vi "Copie de Init_graphe.vi"() -> ()   [LabVIEW 2013]
uses:
  <vilib>/Utility/miscctls.llb/LVRowAndColumnTypeDef.ctl
  <vilib>/Utility/file.llb/Read From Spreadsheet File (string).vi
panel:
  in  "Horodatage":timestamp
  in  "Bouton Aide":bool
  in  "Quit":bool
  out "horodatage_ok":timestamp
  in  "Fichier données":path
  out "Colonne données brutes":string="0"
  out "Ligne données brutes":string="0"
  out "Noms variables":string[](array[string])
  out "Séparateur fichier brute":string
  in  "Valider":bool
  in  "Nouveau format date":bool
  in  "Format d'horodatage":string(combo)="\"%Y-%m-%d %H:%M:%S\""
  in  "Convertir Horodatage":bool
  out "Nb lignes":i32
  in  "Séparateur":u16(ring)=1 items=["", ",", ";", ".", "Tab", "Espace", ":"]
  out "Horodatage_1":timestamp[](array[timestamp]) format="%<%X\n%x>T"
  out "Table":string[][](table)
  out "Donnees":dbl[][](array[numeric])
  in  "Bouton vide 2":bool
  # "Facultatif : \nSélectionner la dernière cellule des noms de variables  en appuyant sur la touche CTRL"
  # "Sélectionner la 1ère cellule\ndes noms de variables"
  # "Sélectionner la 1ère cellule\nd'horodatage"
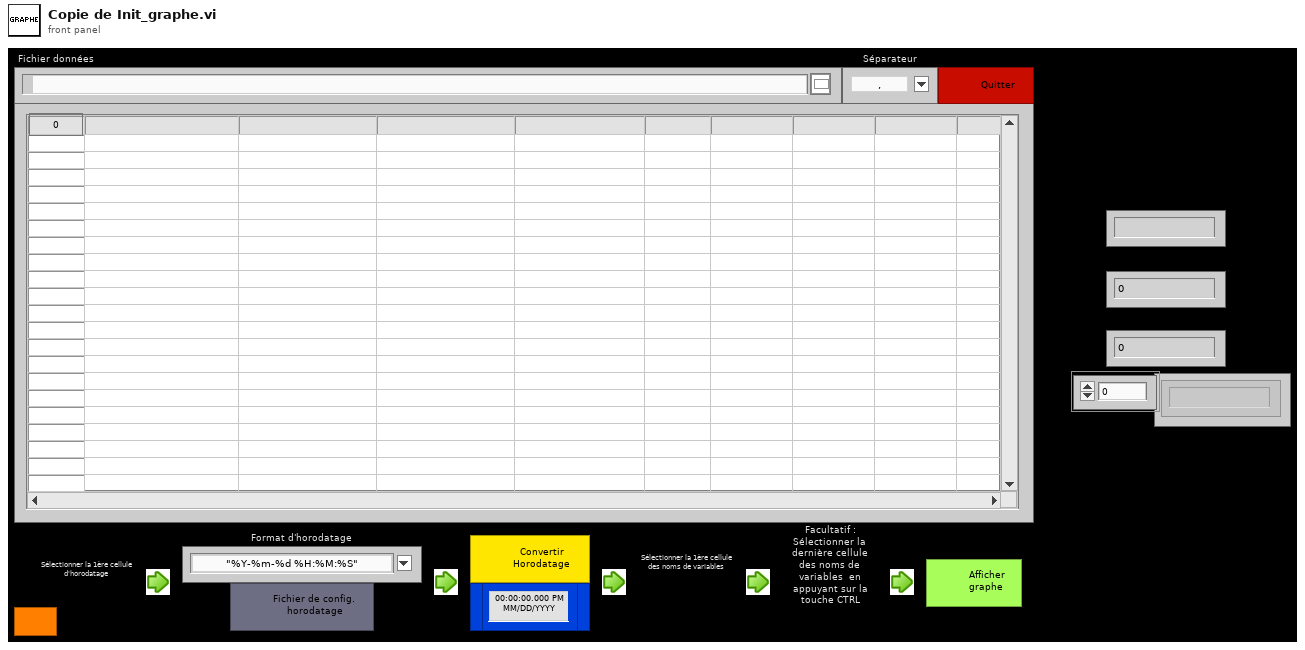
[diagram p1: front panel]
types:
  T1 = typedef "LVRowAndColumnTypeDef.ctl" = cluster{"Row":i32, "Column":i32}
  T2 = typedef "excel Object Reference.ctl" = refnum<k1>
  T3 = enum16{"Left Button", "Center Button", "Right Button", "Window Close"}
  T4 = cluster{"Shift":bool, "Ctrl":bool, "Alt":bool, "Cmd":bool, "Opt":bool}
  T5 = cluster{"Horodatage":timestamp[], "Donnees":dbl[]}[]
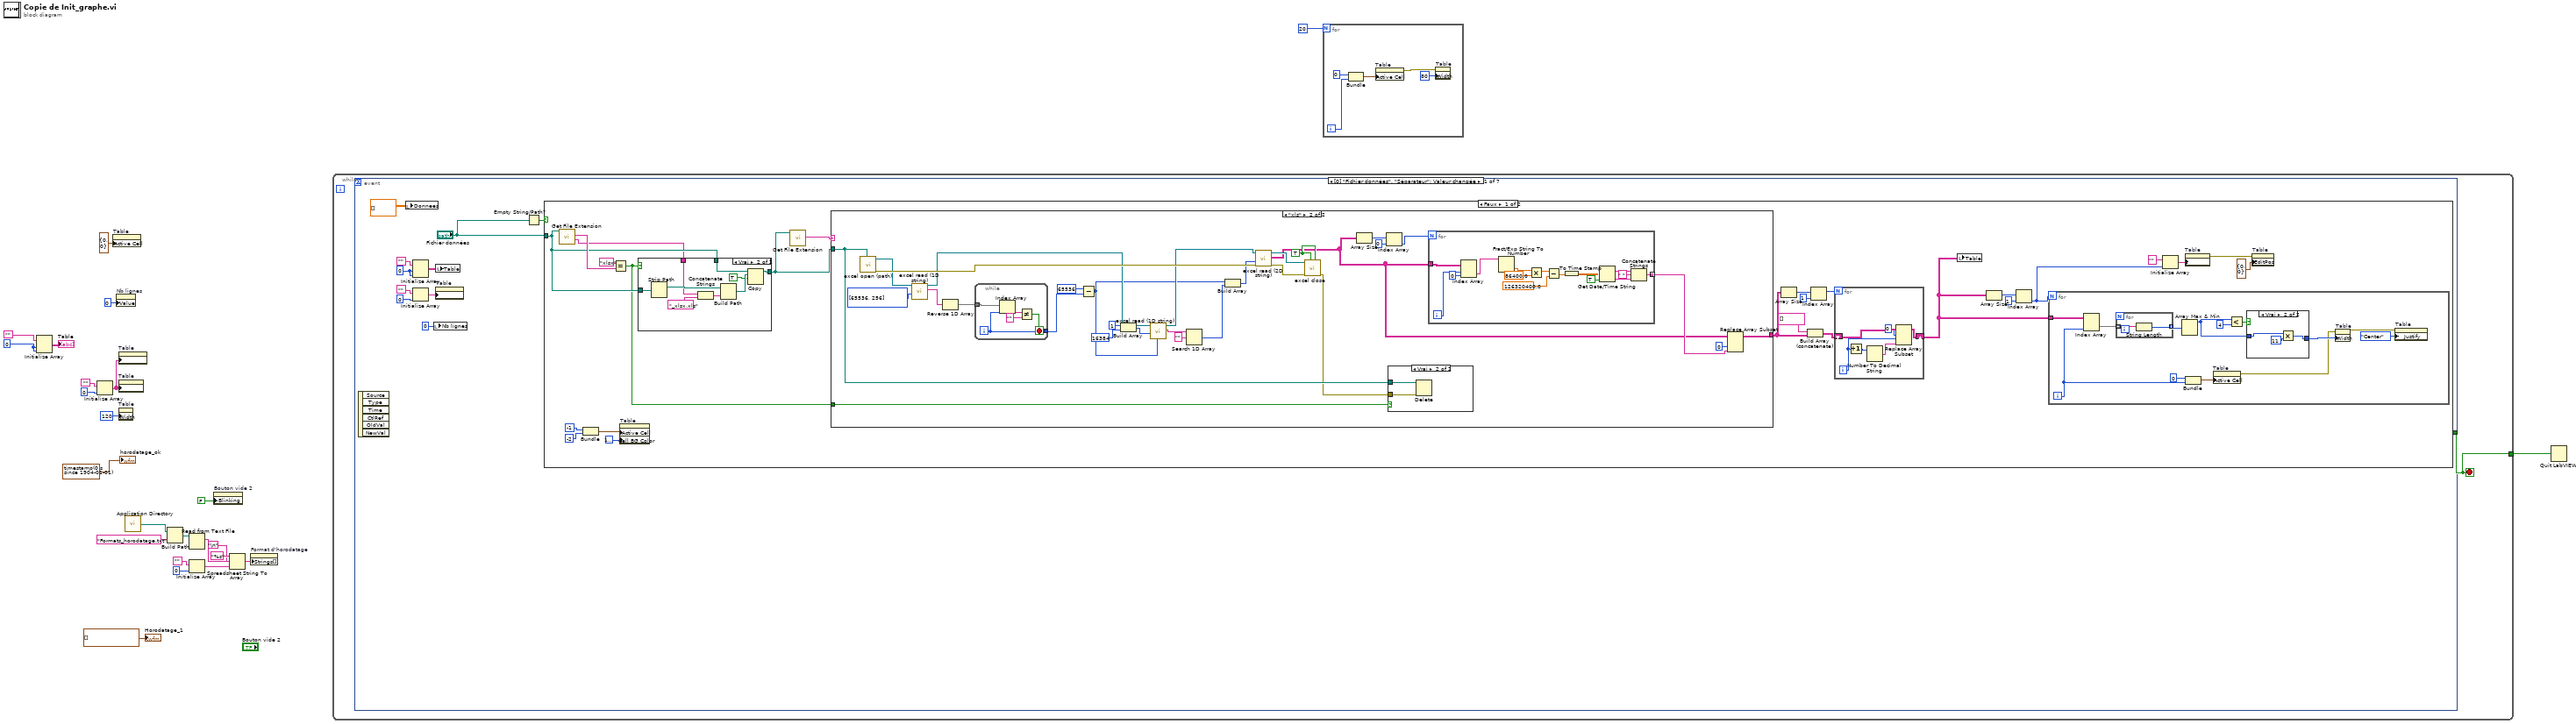
[diagram p0: block diagram]
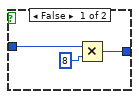
[diagram p3: hidden frame]
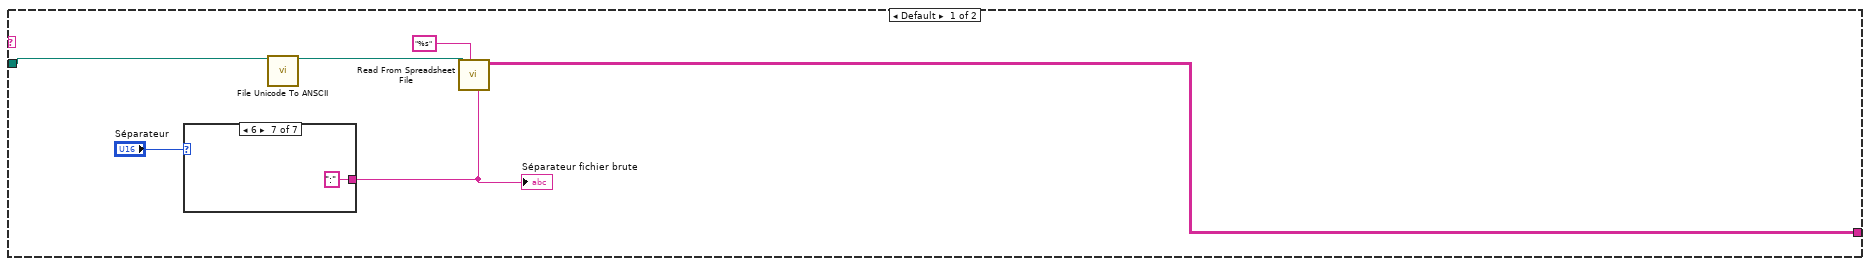
[diagram p4: hidden frame]
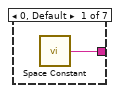
[diagram p5: hidden frame]
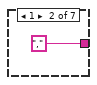
[diagram p6: hidden frame]
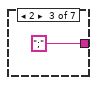
[diagram p7: hidden frame]
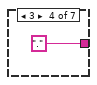
[diagram p8: hidden frame]
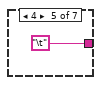
[diagram p9: hidden frame]
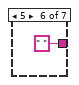
[diagram p10: hidden frame]
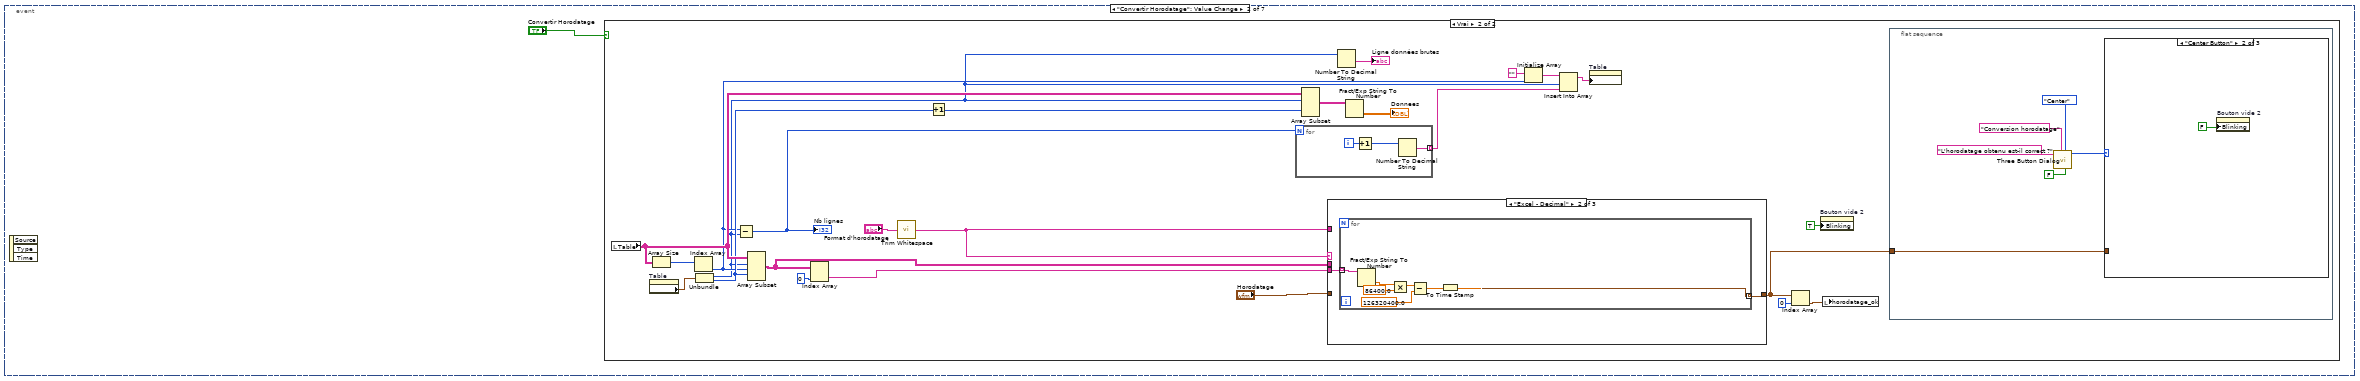
[diagram p13: hidden frame]
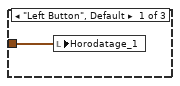
[diagram p15: hidden frame]
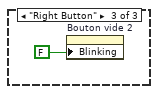
[diagram p16: hidden frame]
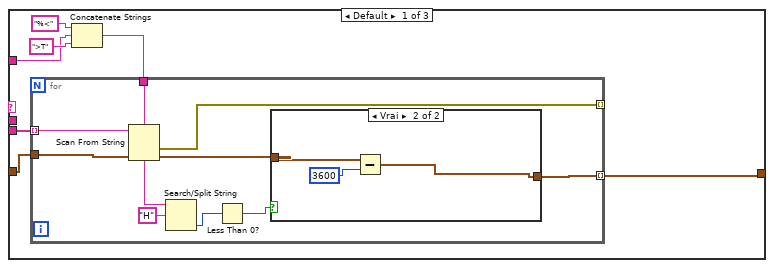
[diagram p17: hidden frame]
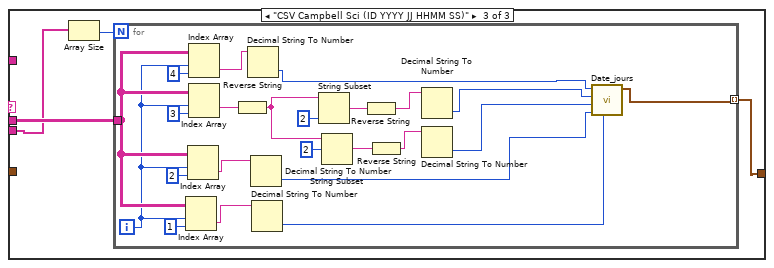
[diagram p19: hidden frame]
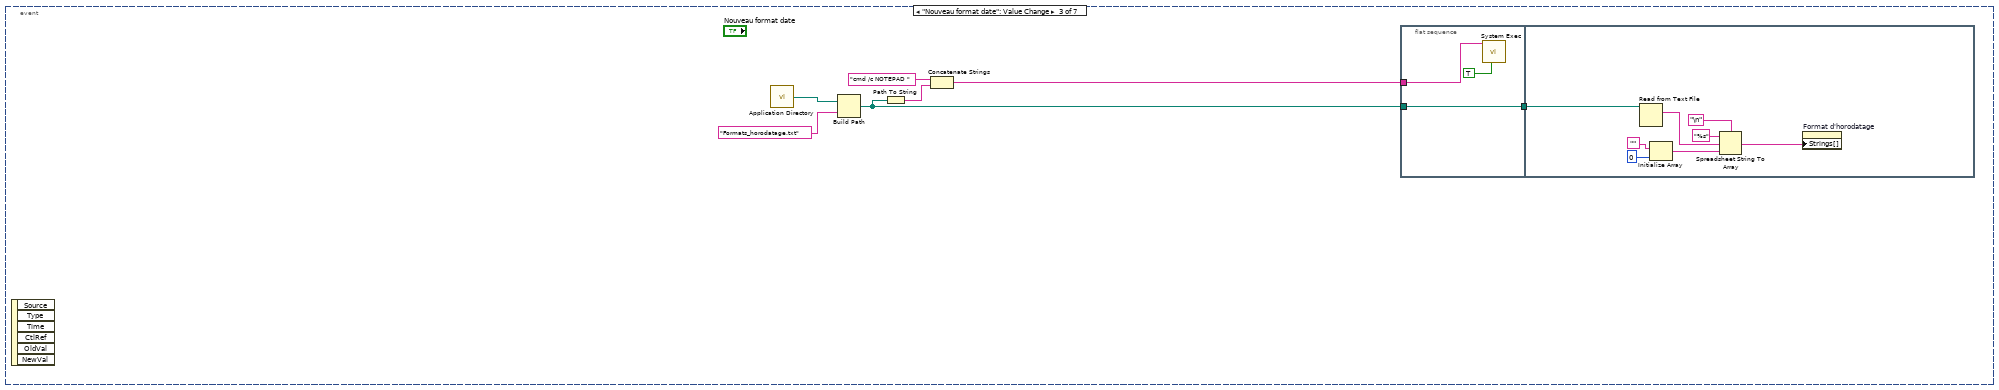
[diagram p20: hidden frame]
diagram:
  w6 = 0 ("taille de la dimension")
  n1 = Initialize Array("", w6, w6) -> (→"Table":string[][])
  n2 = Initialize Array("", 0 ("taille de la dimension")) -> (w13:string[])
  n3 = property on="Table" class="Tbl (strict)"("Active Cell"=T1 {"Row"=0, "Column"=0} ("Cellule active:Cellule active")) -> ()  [unwired: 2 in, 2 out]
  n4 = property on="Nb lignes" class="NumNb (strict)"("Value"=0 ("Nb lignes")) -> ()  [unwired: 2 in, 2 out]
  n5 = property on="Table" class="Tbl (strict)"("Row Headers[]"=w13) -> ()  [unwired: 2 in, 2 out]
  n6 = property on="Table" class="Tbl (strict)"("Column Headers[]"=w13) -> ()  [unwired: 2 in, 2 out]
  n7 = property on="Table" class="Tbl (strict)"("Width"=u32 120 ("Cellule active:Taille de la cellule:Largeur")) -> ()  [unwired: 2 in, 2 out]
  n8 = call <vilib>:"Application Directory.vi"() -> ("Application Directory"=w9:path)
  n9 = Build Path(base path=w9, name or relative path="Formats_horodatage.txt" ("nom ou chemin relatif")) -> (appended path=w17:path)
  n10 = Read from Text File(file (use dialog)=w17) -> (text=w22:string)  [unwired: 3 in, 3 out]
  n11 = Initialize Array("", 0 ("taille de la dimension")) -> (w18:string[])
  n12 = property on="Bouton vide 2" class="Bool"("Blinking"=FALSE ("Clignotant")) -> ()  [unwired: 2 in, 2 out]
  n13 = Spreadsheet String To Array(delimiter (Tab)="\n", format string="%s" ("chaîne de format"), spreadsheet string=w22, array type (2D Dbl)=w18) -> (array=w14:string[])
  n14 = property on="Format d'horodatage" class="ChneDér"("Strings[]"=w14) -> ()  [unwired: 2 in, 2 out]
  n15 = while {
    tunnel: [w25] -> w3
    stop <- w25 stop-if-true
    n16 = event shown="[0] \"Fichier données\", \"Séparateur\": Valeur changée" {
      selector: _ -> [_ _ _ _ _ _ _]
      dyn-events: _ -> [_ _ _ _ _ _ _]
      timeout: _ -> [_ _ _ _ _ _ _]
      tunnel: [_ _ _ _ _ w377 _] -> w25
      event "Fichier données", "Séparateur": Value Change {
        w35 = 0 ("taille de la dimension")
        n17 = event-data() -> ()  [unwired: 1 in, 6 out]
        n18 = local write "Donnees"(dbl[][] [] ("Donnees")) -> ()
        n19 = Initialize Array("", w35, w35) -> (w33:string[][])
        n20 = Initialize Array("", 0 ("taille de la dimension")) -> (w30:string[])
        n21 = local write "Nb lignes"(0 ("Nb lignes")) -> ()
        n22 = local write "Table"(w33) -> ()
        n23 = property on="Table" class="Tbl (strict)"("Row Headers[]"=w30) -> ()  [unwired: 2 in, 2 out]
        n24 = Empty String/Path?(string/path="Fichier données") -> (empty?=w27:bool)
        n25 = case shown="Faux" w27 {
          tunnel: "Fichier données" -> [w40 _]
          frame False {
            n26 = call <vilib>:"Get File Extension.vi"("file"=w40) -> ("filename without extension"=w39:string, "lowercase file extension"=w42:string)  [unwired: 7 in, 2 out]
            n27 = Bundle(-1, -2) -> (w53:cluster{i32, i32})  [unwired: 1 in]
            n28 = Equal?(x="xlsx", y=w42) -> (x = y?=w36:bool)
            n29 = property on="Table" class="Tbl (strict)"("Active Cell"=w53, "Cell BG Color"=u32 16777225) -> ()  [unwired: 2 in, 2 out]
            n30 = case shown="Vrai" w36 {
              tunnel: w40 -> [w61 w70]
              tunnel: [w61 w69] -> w38
              tunnel: w40 -> [_ w67]
              tunnel: w39 -> [_ w64]
              frame False {
              }
              frame True {
                n31 = Strip Path(path=w67) -> (stripped path=w68:path)  [unwired: 1 out]
                n32 = Concatenate Strings(w64, "_xlsx.xls" ("chaîne")) -> (w65:string)
                n33 = Build Path(base path=w68, name or relative path=w65) -> (appended path=w66:path)
                n34 = Copy(9:TRUE ("écraser (F)"), 10:w66, 11:w70) -> (3:w69:path)  [unwired: 2 in, 2 out]
              }
            }
            n35 = call <vilib>:"Get File Extension.vi"("file"=w38) -> ("lowercase file extension"=w37:string)  [unwired: 7 in, 3 out]
            n36 = case shown="\"xls\"" w37 {
              tunnel: w38 -> [w99 w113]
              tunnel: [w101 w114] -> w46
              tunnel: w36 -> [_ w111]
              frame Default {
                n37 = case shown="6" "Séparateur" {
                  tunnel: [w104 "," ";" "." "\t" " " ("String") ":" ("String")] -> w100
                  frame 0, Default {
                    n38 = call <vilib>:"Space Constant.vi"() -> ("String"=w104:string)
                  }
                  frame 1 {
                  }
                  frame 2 {
                  }
                  frame 3 {
                  }
                  frame 4 {
                  }
                  frame 5 {
                  }
                  frame 6 {
                  }
                }
                "Séparateur fichier brute" <- w100
                n39 = call "File Unicode To ANSCII.vi"("file in"=w99) -> ("file out"=w98:path)  [unwired: 18 in]
                n40 = call-poly <vilib>:"Read From Spreadsheet File.vi"("delimiter (\\t)"=w100, "format (%s)"="%s", "file path (dialog if empty)"=w98) -> ("all rows"=w101:string[][])  [unwired: 4 in, 4 out]
              }
              frame "xls" {
                w137 = TRUE ("Override closing behavior")
                n41 = call <userlib>:"excel open (path).vi"("workbook path"=w113) -> ("error out"=w138:errorcluster, "reference"=w136:T2)  [unwired: 9 in]
                n42 = call <userlib>:"excel read (1D string).vi"("array size\n  - #rows\n  - #columns"=i32[] [65536, 256] ("array size\n  - #rows\n  - #columns"), "reference"=w136) -> ("1D String Array"=w134:string[], "duplicate reference"=w127:T2)  [unwired: 7 in, 1 out]
                n43 = Reverse 1D Array(array=w134) -> (reversed array=w132:string[])
                n44 = while {
                  tunnel: w132 -> [w162]
                  tunnel: [w158] -> w131
                  i -> [w158]
                  stop <- w159 stop-if-true
                  n45 = Index Array(array=w162, index=w158) -> (element=w161:string)
                  n46 = Not Equal?(x=w161, y="") -> (x != y?=w159:bool)
                }
                n47 = Subtract(x=65536, y=w131) -> (x-y=w124:i32)
                n48 = Build Array(1 ("élément"), 16384 ("élément")) -> (w128:i32[])
                n49 = call <userlib>:"excel read (1D string).vi"("Row"=w124, "array size\n  - #rows\n  - #columns"=w128, "reference"=w127) -> ("1D String Array"=w123:string[], "duplicate reference"=w126:T2)  [unwired: 6 in, 1 out]
                n50 = Search 1D Array(1D array=w123, element="" ("élément")) -> (index of element=w121:i32)  [unwired: 1 in]
                n51 = Build Array(w124, w121) -> (w133:i32[])
                n52 = call <userlib>:"excel read (2D string).vi"("error in (no error)"=w138, "array size\n  - #rows\n  - #columns"=w133, "reference"=w126) -> ("error out"=w139:errorcluster, "2D String Array"=w115:string[][], "duplicate reference"=w140:T2)  [unwired: 6 in]
                n53 = call <userlib>:"excel close.vi"("Close"=w137, "Override closing behavior"=w137, "error in (no error)"=w139, "reference"=w140) -> ("error out"=w112:errorcluster)  [unwired: 7 in]
                n54 = Array Size(array=w115) -> (size(s)=w117:i32[])
                n55 = Index Array(array=w117, index=0 ("indice")) -> (element=w118:i32)
                n56 = case shown="Vrai" w111 {
                  tunnel: w113 -> [_ w142]
                  tunnel: w112 -> [_ w141]
                  frame False {
                  }
                  frame True {
                    n57 = Delete(path (use dialog)=w142, error in=w141) -> ()  [unwired: 3 in, 3 out]
                  }
                }
                n58 = for {
                  N: w118 -> [_]
                  tunnel: w115 -> [w157]
                  tunnel: [w143] -> w120 mode=indexing
                  i -> [w156]
                  n59 = Index Array(array=w157, index (row)=w156, index (col)=0 ("indice désactivé (col)")) -> (element=w144:string)
                  n60 = Fract/Exp String To Number(string=w144) -> (number=w154:dbl)  [unwired: 3 in, 1 out]
                  n61 = Multiply(x=w154, y=86400.0) -> (x*y=w152:dbl)
                  n62 = Subtract(x=w152, y=126320400.0) -> (x-y=w150:dbl)
                  n63 = To Time Stamp(1:w150) -> (0:w149:timestamp)
                  n64 = Get Date/Time String(seconds (now)=w149, want seconds? (F)=TRUE ("secondes ? (F)")) -> (date string=w147:string, time string=w145:string)  [unwired: 1 in]
                  n65 = Concatenate Strings(w147, " " ("chaîne"), w145) -> (w143:string)
                }
                n66 = Replace Array Subset(array=w115, new element=w120, index (col)=0 ("indice désactivé (col)")) -> (w114:string[][])  [unwired: 1 in]
              }
            }
            n67 = Array Size(array=w46) -> (size(s)=w48:i32[])
            n68 = Build Array (concatenate)(string[] [] ("élément"), w46) -> (w44:string[][])
            n69 = Index Array(array=w48, index=1 ("indice")) -> (element=w47:i32)
            n70 = for {
              N: w47 -> [_]
              shift-right: [w76] -> w50
              shift-left: w44 -> [w75]
              i -> [w72]
              n71 = Increment(x=w72) -> (x+1=w74:i32)
              n72 = Number To Decimal String(number=w74) -> (decimal integer string=w71:string)  [unwired: 1 in]
              n73 = Replace Array Subset(array=w75, new element=w71, index (row)=0 ("indice désactivé (ligne)"), index (col)=w72) -> (w76:string[][])
            }
            n74 = local write "Table"(w50) -> ()
            n75 = Array Size(array=w50) -> (size(s)=w56:i32[])
            n76 = Index Array(array=w56, index=1 ("indice")) -> (element=w43:i32)
            n77 = for {
              N: w43 -> [_]
              tunnel: w50 -> [w89]
              i -> [w83]
              n78 = Index Array(array=w89, index (col)=w83) -> (element=w87:string[])  [unwired: 1 in]
              n79 = for {
                tunnel: w87 -> [w97] mode=indexing
                tunnel: [w96] -> w86 mode=indexing
                n80 = String Length(string=w97) -> (length=w96:i32)
              }
              n81 = Array Max & Min(array=w86) -> (max value=w78:i32)  [unwired: 3 out]
              n82 = Bundle(0, w83) -> (w85:cluster{i32, i32})  [unwired: 1 in]
              n83 = property on="Table" class="Tbl (strict)"("Active Cell"=w85) -> (error out=w84:errorcluster)  [unwired: 2 in, 1 out]
              n84 = Less?(x=w78, y=4) -> (x < y?=w79:bool)
              n85 = case shown="Vrai" w79 {
                tunnel: [w92 w93] -> w88
                tunnel: w78 -> [w90 w94]
                frame False {
                  n86 = Multiply(x=w90, y=8) -> (x*y=w92:i32)
                }
                frame True {
                  n87 = Multiply(x=w94, y=11) -> (x*y=w93:i32)
                }
              }
              n88 = property on="Table" class="Tbl (strict)"(error in=w84, "Width"=w88) -> (error out=w81:errorcluster)  [unwired: 1 in, 1 out]
              n89 = property on="Table" class="Tbl (strict)"(error in=w81, "Justify"=enum16{"Left", "Center", "Right"}."Center" ("Cellule active:Justification de la cellule")) -> ()  [unwired: 1 in, 2 out]
            }
            n90 = Initialize Array("", w43) -> (w59:string[])
            n91 = property on="Table" class="Tbl (strict)"("Column Headers[]"=w59) -> (error out=w57:errorcluster)  [unwired: 2 in, 1 out]
            n92 = property on="Table" class="Tbl (strict)"(error in=w57, "EditPos"=T1 {"Row"=0, "Column"=0} ("Cellule active:Cellule active")) -> ()  [unwired: 1 in, 2 out]
          }
          frame True {
          }
        }
      }
      event "Convertir Horodatage": Value Change {
        n93 = event-data() -> ()  [unwired: 1 in, 3 out]
        n94 = case shown="Vrai" "Convertir Horodatage" {
          frame False {
          }
          frame True {
            n95 = local read "Table"() -> (w183:string[][])
            n96 = property on="Table" class="Tbl (strict)"() -> ("Selection Start"=w186:T1)  [unwired: 2 in, 2 out]
            n97 = Array Size(array=w183) -> (size(s)=w184:i32[])
            n98 = Index Array(array=w184) -> (element=w178:i32)  [unwired: 1 in]
            n99 = Unbundle(w186) -> ("Row"=w174:i32, "Column"=w179:i32)
            n100 = Subtract(x=w178, y=w174) -> (x-y=w169:i32)
            "Nb lignes" <- w169
            n101 = Array Subset(array=w183, index (row)=w174, length (row)=w178, index (col)=w179) -> (w171:string[][])  [unwired: 1 in]
            n102 = Index Array(array=w171, index (col)=0 ("indice (ligne)")) -> (element=w176:string[])  [unwired: 1 in]
            n103 = call <vilib>:"Trim Whitespace.vi"("string"="Format d'horodatage") -> ("trimmed string"=w165:string)  [unwired: 1 in]
            n104 = Increment(x=w179) -> (x+1=w185:i32)
            n105 = for {
              N: w169 -> [_]
              tunnel: [w255] -> w180 mode=indexing
              i -> [w256]
              n106 = Increment(x=w256) -> (x+1=w254:i32)
              n107 = Number To Decimal String(number=w254) -> (decimal integer string=w255:string)  [unwired: 1 in]
            }
            n108 = Array Subset(array=w183, index (row)=w174, index (col)=w185) -> (w187:string[][])  [unwired: 2 in]
            n109 = case shown="\"Excel - Decimal\"" w165 {
              tunnel: "Horodatage" -> [w204 _ _]
              tunnel: w176 -> [w201 w219 w227]
              tunnel: [w200 w218 w229] -> w168
              tunnel: w165 -> [w198 _ _]
              tunnel: w171 -> [_ _ w230]
              frame Default {
                n110 = Concatenate Strings("%<", w198, ">T") -> (w199:string)
                n111 = for {
                  tunnel: [w208] -> w200 mode=indexing
                  tunnel: w204 -> [w213]
                  tunnel: w199 -> [w211]
                  tunnel: w201 -> [w212] mode=indexing
                  tunnel: [w205] -> _ mode=indexing
                  n112 = Scan From String(format string=w211, input string=w212, default 1=w213) -> (error out=w205:errorcluster, output 1=w209:timestamp)  [unwired: 2 in, 2 out]
                  n113 = Search/Split String(string=w211, search string/char (-)="H" ("chaîne/car. recherché (-)")) -> (offset of match=w207:i32)  [unwired: 1 in, 2 out]
                  n114 = Less Than 0?(x=w207) -> (x < 0?=w206:bool)
                  n115 = case shown="Vrai" w206 {
                    tunnel: w209 -> [w214 w217]
                    tunnel: [w214 w215] -> w208
                    frame False {
                    }
                    frame True {
                      n116 = Subtract(x=w217, y=3600) -> (x-y=w215:timestamp)
                    }
                  }
                }
              }
              frame "Excel - Decimal" {
                n117 = for {
                  tunnel: [w220] -> w218 mode=indexing
                  tunnel: w219 -> [w226] mode=indexing
                  n118 = Fract/Exp String To Number(string=w226) -> (number=w225:dbl)  [unwired: 3 in, 1 out]
                  n119 = Multiply(x=w225, y=86400.0) -> (x*y=w223:dbl)
                  n120 = Subtract(x=w223, y=126320400.0) -> (x-y=w221:dbl)
                  n121 = To Time Stamp(1:w221) -> (0:w220:timestamp)
                }
              }
              frame "CSV Campbell Sci (ID YYYY JJ HHMM SS)" {
                n122 = Array Size(array=w227) -> (size(s)=w228:i32)
                n123 = for {
                  N: w228 -> [_]
                  tunnel: w230 -> [w240]
                  tunnel: [w231] -> w229 mode=indexing
                  i -> [w239]
                  n124 = Index Array(array=w240, index (row)=w239, index (col)=1 ("indice désactivé (col)")) -> (element=w237:string)
                  n125 = Index Array(array=w240, index (row)=w239, index (col)=2 ("indice désactivé (col)")) -> (element=w238:string)
                  n126 = Index Array(array=w240, index (row)=w239, index (col)=4 ("indice désactivé (col)")) -> (element=w252:string)
                  n127 = Index Array(array=w240, index (row)=w239, index (col)=3 ("indice désactivé (col)")) -> (element=w250:string)
                  n128 = Reverse String(1:w250) -> (0:w246:string)
                  n129 = Decimal String To Number(string=w252) -> (number=w236:i32)  [unwired: 2 in, 1 out]
                  n130 = Decimal String To Number(string=w238) -> (number=w233:i32)  [unwired: 2 in, 1 out]
                  n131 = Decimal String To Number(string=w237) -> (number=w232:i32)  [unwired: 2 in, 1 out]
                  n132 = String Subset(string=w246, length (rest)=2 ("longueur (reste)")) -> (substring=w248:string)  [unwired: 1 in]
                  n133 = String Subset(string=w246, offset (0)=2) -> (substring=w244:string)  [unwired: 1 in]
                  n134 = Reverse String(1:w248) -> (0:w247:string)
                  n135 = Reverse String(1:w244) -> (0:w243:string)
                  n136 = Decimal String To Number(string=w247) -> (number=w235:i32)  [unwired: 2 in, 1 out]
                  n137 = Decimal String To Number(string=w243) -> (number=w234:i32)  [unwired: 2 in, 1 out]
                  n138 = call "Date_jours.vi"("year"=w232, "jours n"=w233, "hour"=w234, "minute"=w235, "second"=w236) -> ("horodatage"=w231:timestamp)  [unwired: 6 in]
                }
              }
            }
            n139 = Number To Decimal String(number=w174) -> (decimal integer string=→"Ligne données brutes":string)  [unwired: 1 in]
            n140 = Fract/Exp String To Number(string=w187) -> (number=→"Donnees":dbl[][])  [unwired: 3 in, 1 out]
            n141 = Initialize Array("", w178) -> (w181:string[])
            n142 = Insert Into Array(array=w181, index=w174, new element=w180) -> (w170:string[])
            n143 = property on="Table" class="Tbl (strict)"("Row Headers[]"=w170) -> ()  [unwired: 2 in, 2 out]
            n144 = Index Array(array=w168, index=0 ("indice")) -> (element=w167:timestamp)
            n145 = property on="Bouton vide 2" class="Bool"("Blinking"=TRUE ("Clignotant")) -> ()  [unwired: 2 in, 2 out]
            n146 = local write "horodatage_ok"(w167) -> ()
            n147 = flat-sequence {
              tunnel: w168 -> [w189]
              frame #0 {
                n148 = call <vilib>:"Three Button Dialog.vi"("Allow user to close window? (TRUE)"=FALSE, "Justify Message (Left)"=enum16{"Left", "Center", "Right"}."Center", "Window Title (\"\")"="Conversion horodatage" ("error source (\" \")"), "message"="L'horodatage obtenu est-il correct ?" ("error source (\" \")")) -> ("Which Button?"=w192:T3)  [unwired: 7 in]
                n149 = case shown="\"Center Button\"" w192 {
                  tunnel: w189 -> [w195 _ _]
                  frame "Left Button", Default {
                    n150 = local write "Horodatage_1"(w195) -> ()
                  }
                  frame "Center Button" {
                    n151 = property on="Bouton vide 2" class="Bool"("Blinking"=FALSE ("Clignotant")) -> ()  [unwired: 2 in, 2 out]
                  }
                  frame "Right Button" {
                    n152 = property on="Bouton vide 2" class="Bool"("Blinking"=FALSE ("Clignotant")) -> ()  [unwired: 2 in, 2 out]
                  }
                }
              }
            }
          }
        }
      }
      event "Nouveau format date": Value Change {
        n153 = event-data() -> ()  [unwired: 1 in, 6 out]
        n154 = call <vilib>:"Application Directory.vi"() -> ("Application Directory"=w257:path)
        n155 = Build Path(base path=w257, name or relative path="Formats_horodatage.txt" ("nom ou chemin relatif")) -> (appended path=w259:path)
        n156 = Path To String(path=w259) -> (string=w260:string)
        n157 = Concatenate Strings("cmd /c NOTEPAD " ("command line"), w260) -> (w262:string)
        n158 = flat-sequence {
          tunnel: w262 -> [w266]
          tunnel: w259 -> [w264]
          tunnel: [w264] -> w258
          tunnel: w258 -> [w267]
          frame #0 {
            n159 = call <vilib>:"System Exec.vi"("run minimized? (F)"=TRUE, "command line"=w266) -> ()  [unwired: 6 in, 4 out]
          }
          frame #1 {
            n160 = Read from Text File(file (use dialog)=w267) -> (text=w268:string)  [unwired: 3 in, 3 out]
            n161 = Initialize Array("", 0 ("taille de la dimension")) -> (w272:string[])
            n162 = Spreadsheet String To Array(delimiter (Tab)="\n", format string="%s" ("chaîne de format"), spreadsheet string=w268, array type (2D Dbl)=w272) -> (array=w274:string[])
            n163 = property on="Format d'horodatage" class="ChneDér"("Strings[]"=w274) -> ()  [unwired: 2 in, 2 out]
          }
        }
      }
      event "Table": Mouse Down {
        n164 = event-data() -> ("PlatMods"=w282:T4)  [unwired: 1 in, 7 out]
        n165 = local read "Horodatage_1"() -> (w281:timestamp[])
        n166 = property on="Table" class="Tbl (strict)"() -> ("Selection Start"=w277:T1)  [unwired: 2 in, 2 out]
        n167 = Array Size(array=w281) -> (size(s)=w280:i32)
        n168 = Equal To 0?(x=w280) -> (x = 0?=w278:bool)
        n169 = Unbundle(w277) -> ("Column"=w276:i32)  [unwired: 1 out]
        n170 = Equal To 0?(x=w276) -> (x = 0?=w275:bool)
        n171 = Or(x=w275, y=w278) -> (x .or. y?=w279:bool)
        n172 = case shown="Faux" w279 {
          tunnel: w282 -> [w289 _]
          frame False {
            n173 = Unbundle(w289) -> ("Ctrl"=w288:bool)  [unwired: 4 out]
            n174 = case shown="Vrai" w288 {
              tunnel: [w313 w332] -> w285
              tunnel: [w311 w332] -> w284
              frame False {
                n175 = local read "Table"() -> (w310:string[][])
                n176 = property on="Table" class="Tbl (strict)"() -> ("Selection Start"=w312:T1)  [unwired: 2 in, 2 out]
                n177 = Array Size(array=w310) -> (size(s)=w323:i32[])
                n178 = Unbundle(w312) -> ("Row"=w314:i32, "Column"=w316:i32)
                n179 = Index Array(array=w323, index=1 ("indice")) -> (element=w317:i32)
                n180 = Subtract(x=w317, y=w316) -> (x-y=w321:i32)
                n181 = Number To Decimal String(number=w316) -> (decimal integer string=→"Colonne données brutes":string)  [unwired: 1 in]
                n182 = Array Subset(array=w310, index (row)=w314, length (row)=1 ("longueur"), index (col)=w316, length (col)=w321) -> (w324:string[][])
                n183 = Index Array(array=w324, index (row)=0 ("indice (ligne)")) -> (element=w313:string[])  [unwired: 1 in]
                n184 = Initialize Array("", w317) -> (w319:string[])
                n185 = Replace Array Subset(array=w319, new element=w313, index=w316) -> (w311:string[])
                n186 = property on="Table" class="Tbl (strict)"("Column Headers[]"=w311) -> ()  [unwired: 2 in, 2 out]
              }
              frame True {
                n187 = Bundle(-1, -2) -> (w329:cluster{i32, i32})  [unwired: 1 in]
                n188 = property on="Table" class="Tbl (strict)"() -> ("Column Headers[]"=w331:string[], "Selection Start"=w326:T1)  [unwired: 2 in, 2 out]
                n189 = property on="Table" class="Tbl (strict)"("Active Cell"=w329, "Cell BG Color"=u32 16777225) -> ()  [unwired: 2 in, 2 out]
                n190 = Unbundle(w326) -> ("Column"=w333:i32)  [unwired: 1 out]
                n191 = Increment(x=w333) -> (x+1=w335:i32)
                n192 = Array Subset(array=w331, index=0 ("indice"), length=w335) -> (w332:string[])
                n193 = property on="Table" class="Tbl (strict)"("Column Headers[]"=w332) -> ()  [unwired: 2 in, 2 out]
              }
            }
            n194 = for {
              tunnel: w285 -> [w298] mode=indexing
              shift-right: [w300] -> w287
              shift-left: string[] [] -> [w301]
              n195 = Search and Replace String(replace all?=TRUE ("tout remplacer ? (F)"), input string=w298, search string="\"" ("chaîne recherchée"), replace string="" ("chaîne de remplacement (\"\")")) -> (result string=w299:string)  [unwired: 4 in, 3 out]
              n196 = Empty String/Path?(string/path=w299) -> (empty?=w302:bool)
              n197 = case shown="Vrai" w302 {
                tunnel: w301 -> [w308 w309]
                tunnel: [w306 w309] -> w300
                tunnel: w299 -> [w307 _]
                frame False {
                  n198 = Build Array (concatenate)(w308, w307) -> (w306:string[])
                }
                frame True {
                }
              }
            }
            "Noms variables" <- w287
            n199 = for {
              tunnel: w284 -> [w297] mode=indexing
              i -> [w295]
              n200 = Empty String/Path?(string/path=w297) -> (empty?=w293:bool)
              n201 = Bundle(-1, w295) -> (w294:cluster{i32, i32})  [unwired: 1 in]
              n202 = Select(t=u32 16777225, s=w293, f=u32 10473471) -> (s? t:f=w290:u32)
              n203 = property on="Table" class="Tbl (strict)"("Active Cell"=w294, "Cell BG Color"=w290) -> ()  [unwired: 2 in, 2 out]
            }
          }
          frame True {
          }
        }
        n204 = property on="Table" class="Tbl (strict)"("Selection Size"=T1 {"Row"=1, "Column"=1} ("Taille de sélection")) -> ()  [unwired: 2 in, 2 out]
      }
      event "Valider": Value Change {
        n205 = event-data() -> ()  [unwired: 1 in, 6 out]
        n206 = local read "Horodatage_1"() -> (w346:timestamp[])
        n207 = property on="Table" class="Tbl (strict)"() -> ("Column Headers[]"=w341:string[])  [unwired: 2 in, 2 out]
        n208 = Sort 1D Array(array=w341) -> (sorted array=w340:string[])
        n209 = Array Size(array=w346) -> (size(s)=w345:i32)
        n210 = Reverse 1D Array(array=w340) -> (reversed array=w336:string[])
        n211 = Not Equal To 0?(x=w345) -> (x != 0?=w342:bool)
        n212 = Index Array(array=w336) -> (element=w339:string)  [unwired: 1 in]
        n213 = property on="Table" class="Tbl (strict)"("Selection Size"=T1 {"Row"=1, "Column"=1} ("Taille de sélection")) -> ()  [unwired: 2 in, 2 out]
        n214 = Empty String/Path?(string/path=w339) -> (empty?=w338:bool)
        n215 = Not(x=w338) -> (.not. x?=w337:bool)
        n216 = And(x=w337, y=w342) -> (x .and. y?=w343:bool)
        n217 = case shown="Vrai" w343 {
          tunnel: "Valider" -> [_ w354]
          tunnel: w346 -> [_ w353]
          frame False {
            w350 = "" ("Left Button Text (\"Yes\")")
            n218 = call <vilib>:"Three Button Dialog.vi"("Justify Message (Left)"=enum16{"Left", "Center", "Right"}."Center", "Window Title (\"\")"="Problème affichage graphe" ("Window Title (\"\")"), "Right Button Text (\"Cancel\")"=w350, "Center Button Text (\"No\")"="Ok" ("Center Button Text (\"No\")"), "Left Button Text (\"Yes\")"=w350, "message"="Veuillez convertir les dates - heures\net sélectionner au moins une variable\npour afficher le graphe") -> ()  [unwired: 5 in, 1 out]
          }
          frame True {
            n219 = case shown="Vrai" w354 {
              tunnel: w353 -> [_ w360]
              frame False {
              }
              frame True {
                n220 = local read "Table"() -> (w370:string[][])
                n221 = property on="Table" class="Tbl (strict)"() -> ("Selection Start"=w356:T1)  [unwired: 2 in, 2 out]
                n222 = Array Size(array=w370) -> (size(s)=w369:i32[])
                n223 = Unbundle(w356) -> ("Row"=w365:i32, "Column"=w364:i32)
                n224 = Index Array(array=w369, index=1 ("indice")) -> (element=w361:i32)
                n225 = Subtract(x=w361, y=w364) -> (x-y=w367:i32)
                n226 = Array Subset(array=w370, index (row)=w365, length (row)=1 ("longueur"), index (col)=w364, length (col)=w367) -> (w372:string[][])
                n227 = Index Array(array=w372, index (row)=0 ("indice (ligne)")) -> (element=w359:string[])  [unwired: 1 in]
                n228 = Initialize Array("", w361) -> (w363:string[])
                n229 = Replace Array Subset(array=w363, new element=w359, index=w364) -> ()  [unwired: 1 out]
                n230 = local read "Donnees"() -> (w371:dbl[][])
                n231 = property on="Table" class="Tbl (strict)"() -> ("Column Headers[]"=w355:string[])  [unwired: 2 in, 2 out]
                n232 = call "MAJ_Graphe.vi"("Horodatage"=w360, "Donnees"=w371, "Entetes colonnes"=w355) -> ("Graphe"=w358:T5, "Paramètres à afficher"=w357:string[])  [unwired: 5 in]
                n233 = flat-sequence {
                  tunnel: w358 -> [w375]
                  tunnel: w357 -> [w374]
                  frame #0 {
                    n234 = call "Graphe_XY.vi"("Graphe"=w375, "Tableau de chaînes"=w374) -> ()  [unwired: 9 in]
                  }
                  frame #1 {
                    n235 = property on="Table" class="Tbl (strict)"("Active Cell"=T1 {"Row"=0, "Column"=0} ("Cellule active:Cellule active")) -> ()  [unwired: 2 in, 2 out]
                  }
                }
              }
            }
          }
        }
      }
      event "Quit": Value Change {
        n236 = event-data() -> ("NewVal"=w377:bool)  [unwired: 1 in, 5 out]
      }
      event "Bouton Aide": Value Change {
        n237 = event-data() -> ()  [unwired: 1 in, 6 out]
        n238 = call <vilib>:"Application Directory.vi"() -> ("Application Directory"=w379:path)
        n239 = Build Path(base path=w379, name or relative path="Logiciel GRAPHE_Instruction.pdf" ("standard input")) -> (appended path=w378:path)
        n240 = call "Open PDF.vi"("Path"=w378) -> ()  [unwired: 5 in, 2 out]
      }
    }
  }
  n241 = for {
    N: 20 -> [_]
    i -> [w383]
    n242 = Bundle(0, w383) -> (w384:cluster{i32, i32})  [unwired: 1 in]
    n243 = property on="Table" class="Tbl (strict)"("Active Cell"=w384) -> (error out=w381:errorcluster)  [unwired: 2 in, 1 out]
    n244 = property on="Table" class="Tbl (strict)"(error in=w381, "Width"=u32 80 ("Cellule active:Taille de la cellule:Largeur")) -> ()  [unwired: 1 in, 2 out]
  }
  n245 = Quit LabVIEW(quit? (T)=w3) -> ()
  "Horodatage_1" <- timestamp[] [] ("Horodatage")
  "horodatage_ok" <- timestamp(0 s since 1904-01-01)
